vi "GenArrBySTD.vi"(8 "2D Array":dbl[][](array[numeric]), 11 "Last idx -":i32) -> (0 "Std By This Row":i32, 1 "This Idx":u64, 2 "2D ResUArr":u64[][](array[numeric]), 3 "1D ResUArr":u64[](array[numeric]))   [LabVIEW 2023]
panel:
  out "StdRes":i32
  out "Size":i32
  out "Attempts":i32
  out "Check":dbl[](array[numeric]) format="%#_4g"
  # "Генерирай масив от уникални числа(само в реда),\nкоито имат същото Std каквото има реда \nс индекс idx от масива с официалните резултати."
  # "="
  # "-"
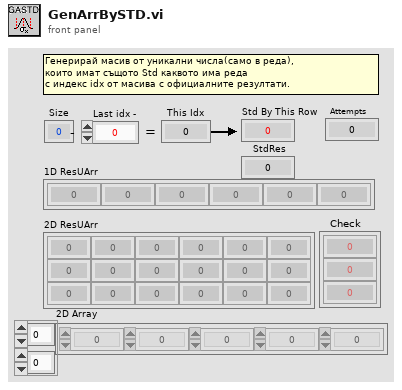
[diagram p1: front panel]
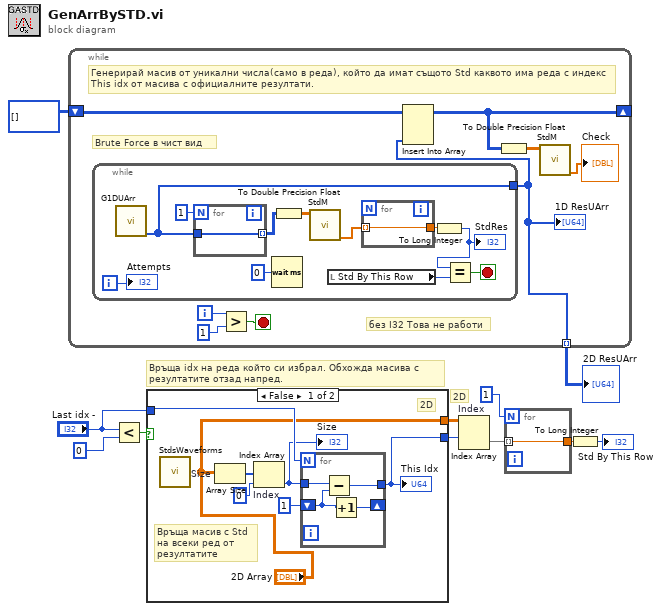
[diagram p0: block diagram]
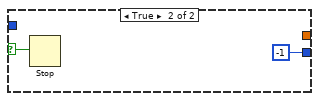
[diagram p2: hidden frame]
diagram:
  # "2D"
  # "Връща idx на реда който си избрал. Обхожда масива с\nрезултатите отзад напред."
  n1 = while {
    tunnel: [w16] -> w3 mode=indexing
    shift-right: [w14] -> _
    shift-left: u64[][] [] -> [w15]
    i -> [w17]
    stop <- w18 stop-if-true
    # "без I32 Това не работи"
    # "Brute Force в чист вид"
    # "Генерирай масив от уникални числа(само в реда), който да имат същото Std каквото има реда с индекс This idx от масива с официалните резултати."
    n2 = while {
      tunnel: [w27] -> w16
      i -> [w24]
      stop <- w28 stop-if-true
      n3 = call "G1DUArr.vi"() -> ("1D UArr"=w27:u64[])  [unwired: 11 in]
      n4 = for {
        N: 1 -> [_]
        tunnel: w27 -> [w32]
        tunnel: [w32] -> w26 mode=indexing
      }
      n5 = Wait (ms)(milliseconds to wait=u32 0) -> ()  [unwired: 1 out]
      n6 = To Double Precision Float(number=w26) -> (double precision float=w23:dbl[][])
      n7 = call "StdM.vi"("2D"=w23) -> ("1D Std"=w25:dbl[])  [unwired: 6 in, 4 out]
      n8 = local read "Std By This Row"() -> (w29:i32)
      n9 = for {
        tunnel: w25 -> [w31] mode=indexing
        tunnel: [w31] -> w22
      }
      n10 = To Long Integer(number=w22) -> (32bit integer=w20:i32)
      "StdRes" <- w20
      n11 = Equal?(x=w20, y=w29) -> (x = y?=w28:bool)
      "Attempts" <- w24
    }
    "1D ResUArr" <- w16
    n12 = Greater?(x=w17, y=1) -> (0:w18:bool)
    n13 = Insert Into Array(array=w15, new element=w16) -> (w14:u64[][])  [unwired: 2 in]
    n14 = To Double Precision Float(number=w14) -> (double precision float=w12:dbl[][])
    n15 = call "StdM.vi"("2D"=w12) -> ("1D Std"=→"Check":dbl[])  [unwired: 6 in, 4 out]
  }
  "2D ResUArr" <- w3
  n16 = Less?(x="Last idx -", y=0) -> (x < y?=w10:bool)
  n17 = case shown="False" w10 {
    selector: w10 -> [_ w45]
    tunnel: "Last idx -" -> [w37 _]
    tunnel: [w36 -1] -> w8
    tunnel: ["2D Array" _] -> w7
    frame False {
      # "2D"
      # "Връща масив с Std \nна всеки ред от \nрезултатите"
      n18 = call "StdsWaveforms.vi"() -> ()  [unwired: 9 in, 3 out]
      n19 = Array Size "Size"(array="2D Array") -> (size(s)=w39:i32[])
      n20 = Index Array "Index"(array=w39, index=0) -> (element=w34:i32)
      "Size" <- w34
      n21 = for {
        N: w37 -> [_]
        shift-right: [w41] -> _
        shift-left: u64 1 -> [w42]
        tunnel: w34 -> [w43]
        tunnel: [w40] -> w36
        n22 = Subtract(x=w43, y=w42) -> (x-y=w40:u64)
        n23 = Increment(x=w42) -> (x+1=w41:u64)
      }
      "This Idx" <- w36
    }
    frame True {
      n24 = Stop(stop? (T)=w45) -> ()
    }
  }
  n25 = Index Array "Index"(array=w7, index (row)=w8) -> (element=w6:dbl[])  [unwired: 1 in]
  n26 = for {
    N: 1 -> [_]
    tunnel: w6 -> [w46] mode=indexing
    tunnel: [w46] -> w4
  }
  n27 = To Long Integer(number=w4) -> (32bit integer=→"Std By This Row":i32)
